vi "file - read-write - list of lines.vi"(7 "read/write control":T1, 9 "header":string, 10 "list of lines IN":string[](array[string]), 11 "file path":path=path "\\\\rus-one\\newdata/data/Ultrasound/Experiment/ProbeTest/Probe10/Hg1201-6-C185-550Cair-3c-83K/sweep3/9w/3366_a.dat") -> (1 "header OUT":string, 2 "list of lines OUT":string[](array[string]))   [LabVIEW 2018]
uses:
  file -- read-write control.ctl
  <vilib>/Utility/file.llb/Write Delimited Spreadsheet (string).vi
  <vilib>/Utility/file.llb/Read Delimited Spreadsheet (string).vi
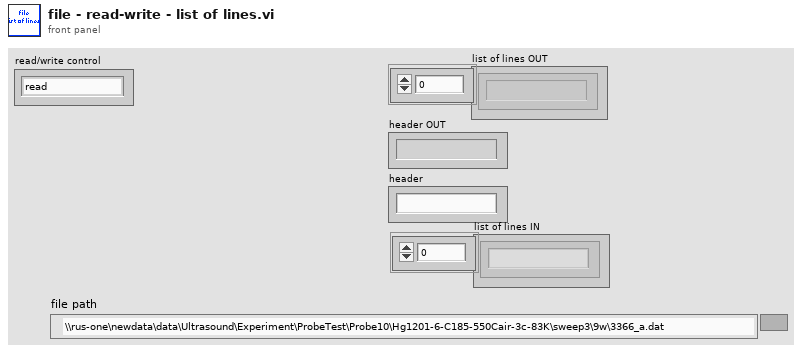
[diagram p1: front panel]
types:
  T1 = typedef "file -- read-write control.ctl" = enum16{"read", "write all", "append one line"}
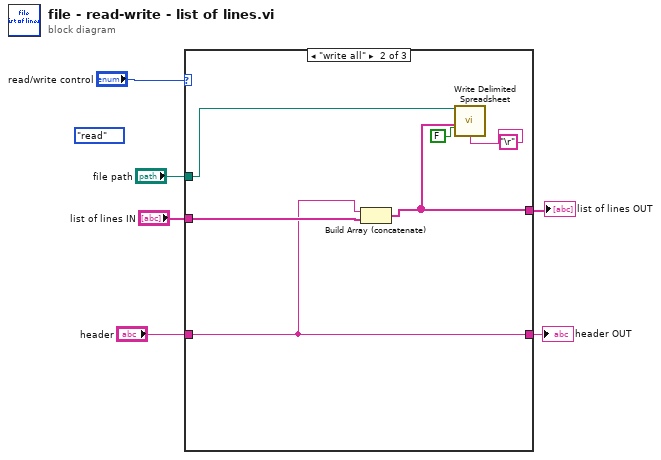
[diagram p0: block diagram]
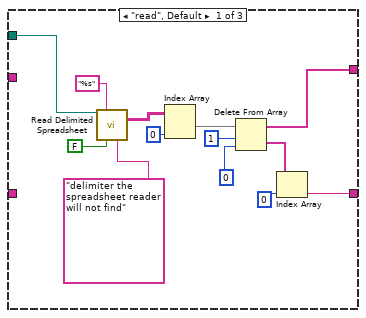
[diagram p2: hidden frame]
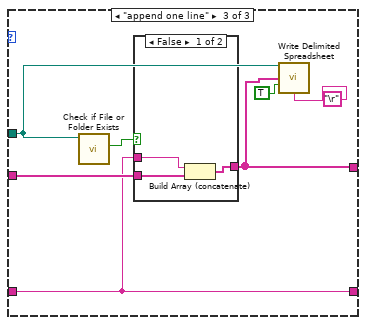
[diagram p3: hidden frame]
diagram:
  (unwired) file_--_read-write_control."read" ("read/write control")
  n1 = case shown="\"write all\"" "read/write control" {
    tunnel: "file path" -> [w12 w23 w29]
    tunnel: [w8 w20 w26] -> w5
    tunnel: [w7 w21 w27] -> w4
    tunnel: "header" -> [_ w21 w27]
    tunnel: "list of lines IN" -> [_ w22 w28]
    frame "read", Default {
      n2 = call-poly <vilib>:"Read Delimited Spreadsheet.vi"("file path (dialog if empty)"=w12, "format (%s)"="%s", "transpose? (F)"=FALSE ("append to file? (new file:F)"), "delimiter (\\t)"="delimiter the spreadsheet reader will not find" ("delimiter (\\t)")) -> ("all rows"=w17:string[][])  [unwired: 6 in, 5 out]
      n3 = Index Array(array=w17, index (col)=0 ("disabled index (col)")) -> (element=w15:string[])  [unwired: 1 in]
      n4 = Delete From Array(array=w15, length=1, index=0) -> (deleted portion=w10:string[], array with subset deleted=w8:string[])
      n5 = Index Array(array=w10, index=0 ("disabled index (col)")) -> (element=w7:string)
    }
    frame "write all" {
      n6 = Build Array (concatenate)(w21, w22) -> (w20:string[])
      n7 = call-poly <vilib>:"Write Delimited Spreadsheet.vi"("file path (dialog if empty)"=w23, "1D data"=w20, "append to file? (new file:F)"=FALSE, "delimiter (\\t)"="\r") -> ()  [unwired: 10 in, 2 out]
    }
    frame "append one line" {
      n8 = call <vilib>:"Check if File or Folder Exists.vi"("path"=w29) -> ("file or folder exists?"=w30:bool)  [unwired: 8 in, 2 out]
      n9 = case shown="False" w30 {
        tunnel: w28 -> [w35 w36]
        tunnel: w27 -> [w34 _]
        tunnel: [w33 w36] -> w26
        frame False {
          n10 = Build Array (concatenate)(w34, w35) -> (w33:string[])
        }
        frame True {
        }
      }
      n11 = call-poly <vilib>:"Write Delimited Spreadsheet.vi"("file path (dialog if empty)"=w29, "1D data"=w26, "append to file? (new file:F)"=TRUE, "delimiter (\\t)"="\r") -> ()  [unwired: 10 in, 2 out]
    }
  }
  "list of lines OUT" <- w5
  "header OUT" <- w4
